vi "Histogram_Automatic.vi"(4 "Properties":T2={"Color"=2147483647, "Cumulative"=FALSE, "Normalize"=FALSE, "Line"={"Style"=enum."Automatic", "Color"=2147483647, "Width"=nan}, "Display"={"Alpha"=nan, "Z Order"=nan}} {"Line"."Color" items=["Automatic"=2147483647, "Black"=0, "White"=16777215, "Red"=16711680, "Green"=2263842, "Blue"=255, "Cyan"=65535, "Magenta"=16711935, "Yellow"=16776960]; "Color" items=["Automatic"=2147483647, "Black"=0, "White"=16777215, "Red"=16711680, "Green"=2263842, "Blue"=255, "Cyan"=65535, "Magenta"=16711935, "Yellow"=16776960]}, 5 "Data Range":T1={"Data Min"=nan, "Data Max"=nan}, 6 "Legend Title":string, 7 "Bins":i32=-1, 8 "error in (no error)":errorcluster, 10 "Data":dbl[](array[numeric]), 11 "Plot ID":T7 format="%x") -> (0 "error out":errorcluster, 3 "Plot ID Out":T7 format="%x")   [LabVIEW 2013, in "Advanced Plotting Toolkit.lvlib"]
doc: "Create a 1D histogram bar plot from an array of data."
uses:
  Advanced Plotting Toolkit.lvlib
  typedefs/PlotID.ctl
  HistogramProperties.ctl
  typedefs/PlotColor.ctl
  properties/Line.ctl
  properties/Line_Style.ctl
  properties/Display.ctl
  HistogramRange.ctl
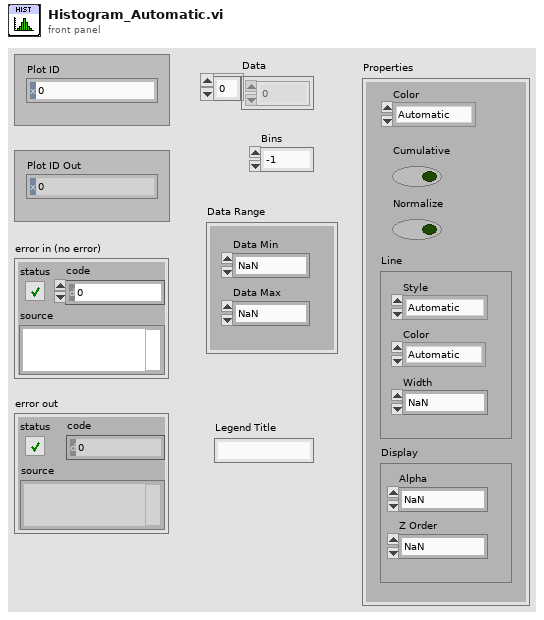
[diagram p1: front panel]
types:
  T1 = typedef "Advanced Plotting Toolkit.lvlib/HistogramRange.ctl" = cluster{"Data Min":dbl, "Data Max":dbl}
  T2 = typedef "Advanced Plotting Toolkit.lvlib/HistogramProperties.ctl" = cluster{"Color":T3, "Cumulative":bool, "Normalize":bool, "Line":T4, "Display":T6}
  T3 = typedef "Advanced Plotting Toolkit.lvlib/PlotColor.ctl" = u32
  T4 = typedef "Advanced Plotting Toolkit.lvlib/Line.ctl" = cluster{"Style":T5, "Color":T3, "Width":sgl}
  T5 = typedef "Advanced Plotting Toolkit.lvlib/Line_Style.ctl" = enum16{"Automatic", "Solid", "Dashed", "Dotted", "Dash-dot", "Invisible"}
  T6 = typedef "Advanced Plotting Toolkit.lvlib/Display.ctl" = cluster{"Alpha":dbl, "Z Order":dbl}
  T7 = typedef "Advanced Plotting Toolkit.lvlib/PlotID.ctl" = i32
  T8 = typedef "Advanced Plotting Toolkit.lvlib/KeyValue.ctl" = cluster{"Key":string, "Value":string}
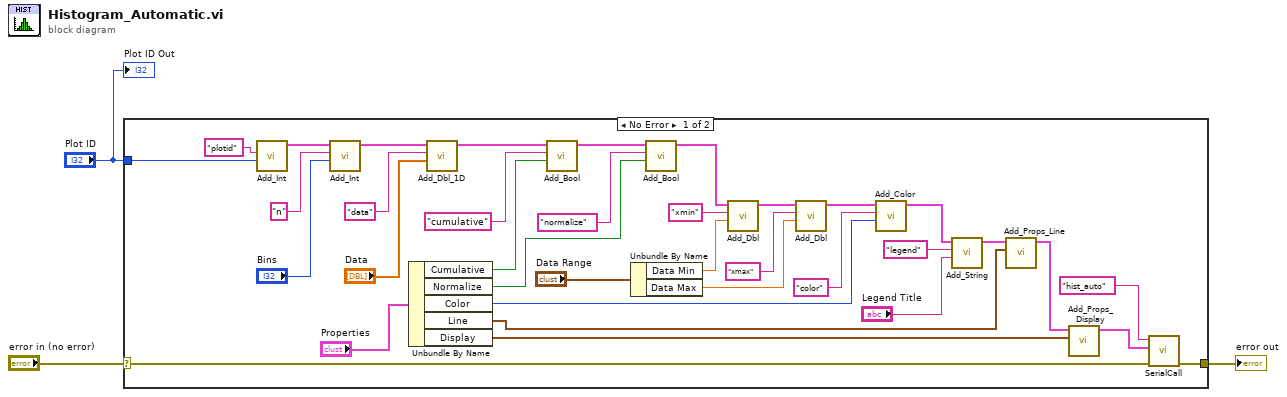
[diagram p0: block diagram]
diagram:
  n1 = case shown="No Error" "error in (no error)" {
    selector: "error in (no error)" -> [w29 w40]
    tunnel: "Plot ID" -> [w39 _]
    tunnel: [w28 w40] -> w1
    frame No Error {
      n2 = call "Add_Int.vi"("Value"=w39, "Key"="plotid") -> ("Keyword Array Out"=w35:T8[])  [unwired: 9 in]
      n3 = call "Add_Int.vi"("Value"="Bins", "Key"="n", "Keyword Array"=w35) -> ("Keyword Array Out"=w34:T8[])  [unwired: 8 in]
      n4 = Unbundle By Name("Properties") -> ("Cumulative"=w25:bool, "Normalize"=w24:bool, "Color"=w18:T3, "Line"=w12:T4, "Display"=w10:T6)
      n5 = call "Add_Dbl_1D.vi"("Value"="Data", "Key"="data", "Keyword Array"=w34) -> ("Keyword Array Out"=w8:T8[])  [unwired: 8 in]
      n6 = call "Add_Bool.vi"("Value"=w25, "Key"="cumulative", "Keyword Array"=w8) -> ("Keyword Array Out"=w21:T8[])  [unwired: 8 in]
      n7 = Unbundle By Name("Data Range") -> ("Data Min"=w14:dbl, "Data Max"=w13:dbl)
      n8 = call "Add_Bool.vi"("Value"=w24, "Key"="normalize", "Keyword Array"=w21) -> ("Keyword Array Out"=w20:T8[])  [unwired: 8 in]
      n9 = call "Add_Dbl.vi"("Value"=w14, "Key"="xmin", "Keyword Array"=w20) -> ("Keyword Array Out"=w19:T8[])  [unwired: 8 in]
      n10 = call "Add_Dbl.vi"("Value"=w13, "Key"="xmax", "Keyword Array"=w19) -> ("Keyword Array Out"=w16:T8[])  [unwired: 8 in]
      n11 = call "Add_Color.vi"("Color"=w18, "Key"="color", "Keyword Array"=w16) -> ("Keyword Array Out"=w7:T8[])  [unwired: 8 in]
      n12 = call "Add_String.vi"("Value"="Legend Title", "Key"="legend", "Keyword Array"=w7) -> ("Keyword Array Out"=w6:T8[])  [unwired: 8 in]
      n13 = call "Add_Props_Line.vi"("Line"=w12, "Keyword Array"=w6) -> ("Keyword Array Out"=w11:T8[])  [unwired: 9 in]
      n14 = call "Add_Props_Display.vi"("Display"=w10, "Keyword Array"=w11) -> ("Keyword Array Out"=w9:T8[])  [unwired: 9 in]
      n15 = call "SerialCall.vi"("error in (no error)"=w29, "data"=w9, "Resource"="hist_auto") -> ("error out"=w28:errorcluster)  [unwired: 7 in, 1 out]
    }
    frame Error {
    }
  }
  "error out" <- w1
  "Plot ID Out" <- "Plot ID"
